vi "Write Spectrum Analyzer.lvclass.vi"(10 "Spectrum Analyzer.lvclass":refnum<class "Spectrum Analyzer.lvclass">, 11 "AM-AM in":refnum<class "AM-AM.lvclass">) -> (3 "AM-AM out":refnum<class "AM-AM.lvclass">)   [LabVIEW 2020, in "AM-AM.lvclass"]
uses:
  AM-AM.lvclass
  Instruments/Spectrum Analyzer/Spectrum Analyzer.lvclass
  AM-AM.lvclass/AM-AM.ctl
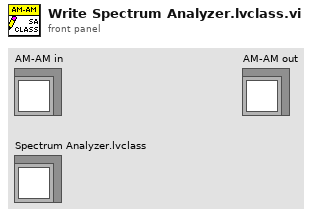
[diagram p1: front panel]
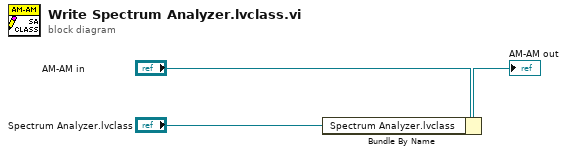
[diagram p0: block diagram]
diagram:
  n1 = Bundle By Name(cluster="AM-AM in", "Spectrum Analyzer.lvclass"="Spectrum Analyzer.lvclass") -> (→"AM-AM out":refnum<class "AM-AM.lvclass">)
